vi "data create.vi"(8 "old":string[](array[string]), 9 "y 2":dbl=0.025 format="%#_13g", 10 "索引":i32=1, 11 "new":string[](array[string])) -> (3 "Data":string)   [LabVIEW 2015]
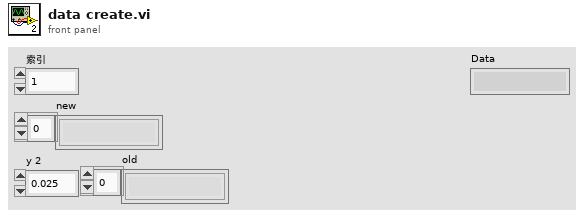
[diagram p1: front panel]
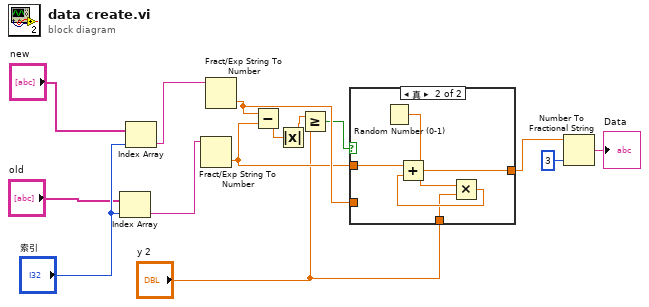
[diagram p0: block diagram]
diagram:
  n1 = Index Array(array="old", index="索引") -> (element=w10:string)
  n2 = Index Array(array="new", index="索引") -> (element=w7:string)
  n3 = Fract/Exp String To Number(string=w10) -> (number=w13:dbl)  [unwired: 3 in, 1 out]
  n4 = Fract/Exp String To Number(string=w7) -> (number=w14:dbl)  [unwired: 3 in, 1 out]
  n5 = Subtract(x=w14, y=w13) -> (x-y=w2:dbl)
  n6 = Absolute Value(x=w2) -> (abs(x)=w1:dbl)
  n7 = Greater Or Equal?(x=w1, y="y 2") -> (x >= y?=w12:bool)
  n8 = case shown="真" w12 {
    tunnel: w13 -> [_ w20]
    tunnel: w14 -> [w15 _]
    tunnel: [w15 w17] -> w8
    tunnel: "y 2" -> [_ w16]
    frame False {
    }
    frame True {
      n9 = Random Number (0-1)() -> (number: 0 to 1=w19:dbl)
      n10 = Multiply(x=w19, y=w16) -> (x*y=w18:dbl)
      n11 = Add(x=w20, y=w18) -> (x+y=w17:dbl)
    }
  }
  n12 = Number To Fractional String(number=w8, precision (6)=i16 3 ("精度(6)")) -> (F-format string=→"Data":string)  [unwired: 2 in]
